vi "RF_calibration_NF_WF1974_scan.vi"() -> ()   [LabVIEW 2017]
uses:
  instr.lib/Tektronix TDS 200 1000 2000 Series/Tektronix TDS 200 1000 2000 Series.lvlib
  instr.lib/Keithley 3390/Keithley 3390.lvlib
panel:
  out "Graph 3":cluster{dbl[], dbl[]}(graph)={[200.0, 300.0, 300.0, 300.0, 300.0], [0.0544000007, 0.0544000007, 0.0903999954, 0.0903999954, 0.1011999995]}
  in  "COMMENT":string="TEST"
  out "Graph 2":cluster{dbl[], dbl[]}(graph)={[200.0, 300.0, 300.0, 300.0, 300.0], [1200.0, 1200.0, 2000.0, 2000.0, 2400.0]}
  out "Graph":cluster{dbl[], dbl[]}(graph)={[200.0, 300.0, 300.0, 300.0, 300.0], [160000.0, 160000.0, 160000.0, 160000.0, 160000.0]}
  in  "Tab Control":enum32{"CONFIG", "MAIN", "DIAGNOSIS"}(tab)
  in  "WF1974":refnum<visa-resource-name>="USB0::0x0D4A::0x000E::9260521::INSTR"
  in  "Columns":string[](array[string])=["SF1/SF2", "l (mm)", "FG freq (Hz)", "FG V (mVpp)", "CH1 Monitor (Vpp)", "CH2 VR (Vpp)", "CH2 Antenna (Vpp)"]
  in  "File path":path=path "C:/LabVIEW/DATA/J-PARC_202206/RF_zscans"
  in  "Tektronix":refnum<visa-resource-name>="USB0::0x0699::0x0365::C035183::INSTR"
  out "File ref (calibration)":refnum<file>
  out "Error Out":errorcluster={"status"=FALSE, "code"=1073676290, "source"="NF WF1973_74 Initialize.vi->RF_calibration_NF_WF1974_scan.vi内のVISAイベント有効"}
  in  "Measure":bool
  in  "Vamp lower lim":dbl=0.4 format="%_4f"
  in  "Vamp upper lim":dbl=3000.0 format="%_4f"
  in  "FG reset":bool
  in  "Amplitude (mVpp)":dbl=1200.0 format="%_6f"
  in  "FG Output":bool
  in  "Frequency (Hz)":dbl=160000.0 format="%_8e"
  out "Measurement index":i32
  out "CH 1 measurement":dbl=0.1011999995 format="%_6g"
  out "CH 2 measurement":dbl=3.4600000381 format="%_6g"
  out "CH3 measurement":dbl=0.00208
  in  "L (mm)":dbl=300.0
  in  "SF1 or2?":u32=1
  out "Latest measurements":dbl[][](array[numeric]) format="%_4e"
  out "index":i32[](array[numeric])
  out "error out (Agilent)":errorcluster
  out "error out (Tektronix)":errorcluster
  out "error out (file operation)":errorcluster
  in  "STOP":bool
  # "Z SCAN OF THE RF FIELD"
  # "SCAN INPUTS"
  # "FG CONTROL"
  # "TEKTRONIX READOUT"
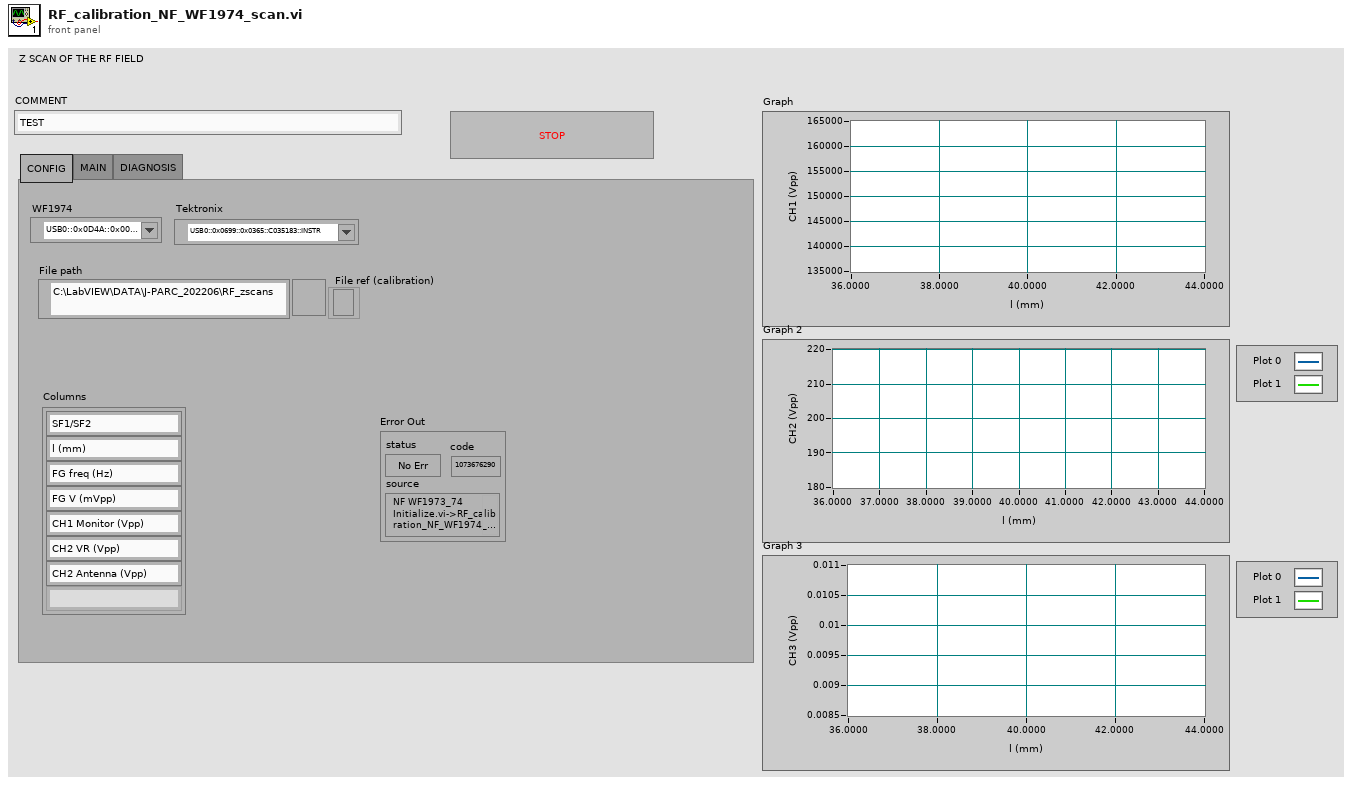
[diagram p1: front panel]
types:
  T1 = cluster{"Baud Rate":u32, "Parity":u16, "Stop Bits":u16, "Flow Control":u16}
  T2 = enum16{"open", "replace", "create", "open or create", "replace or create", "replace or create with confirmation"}
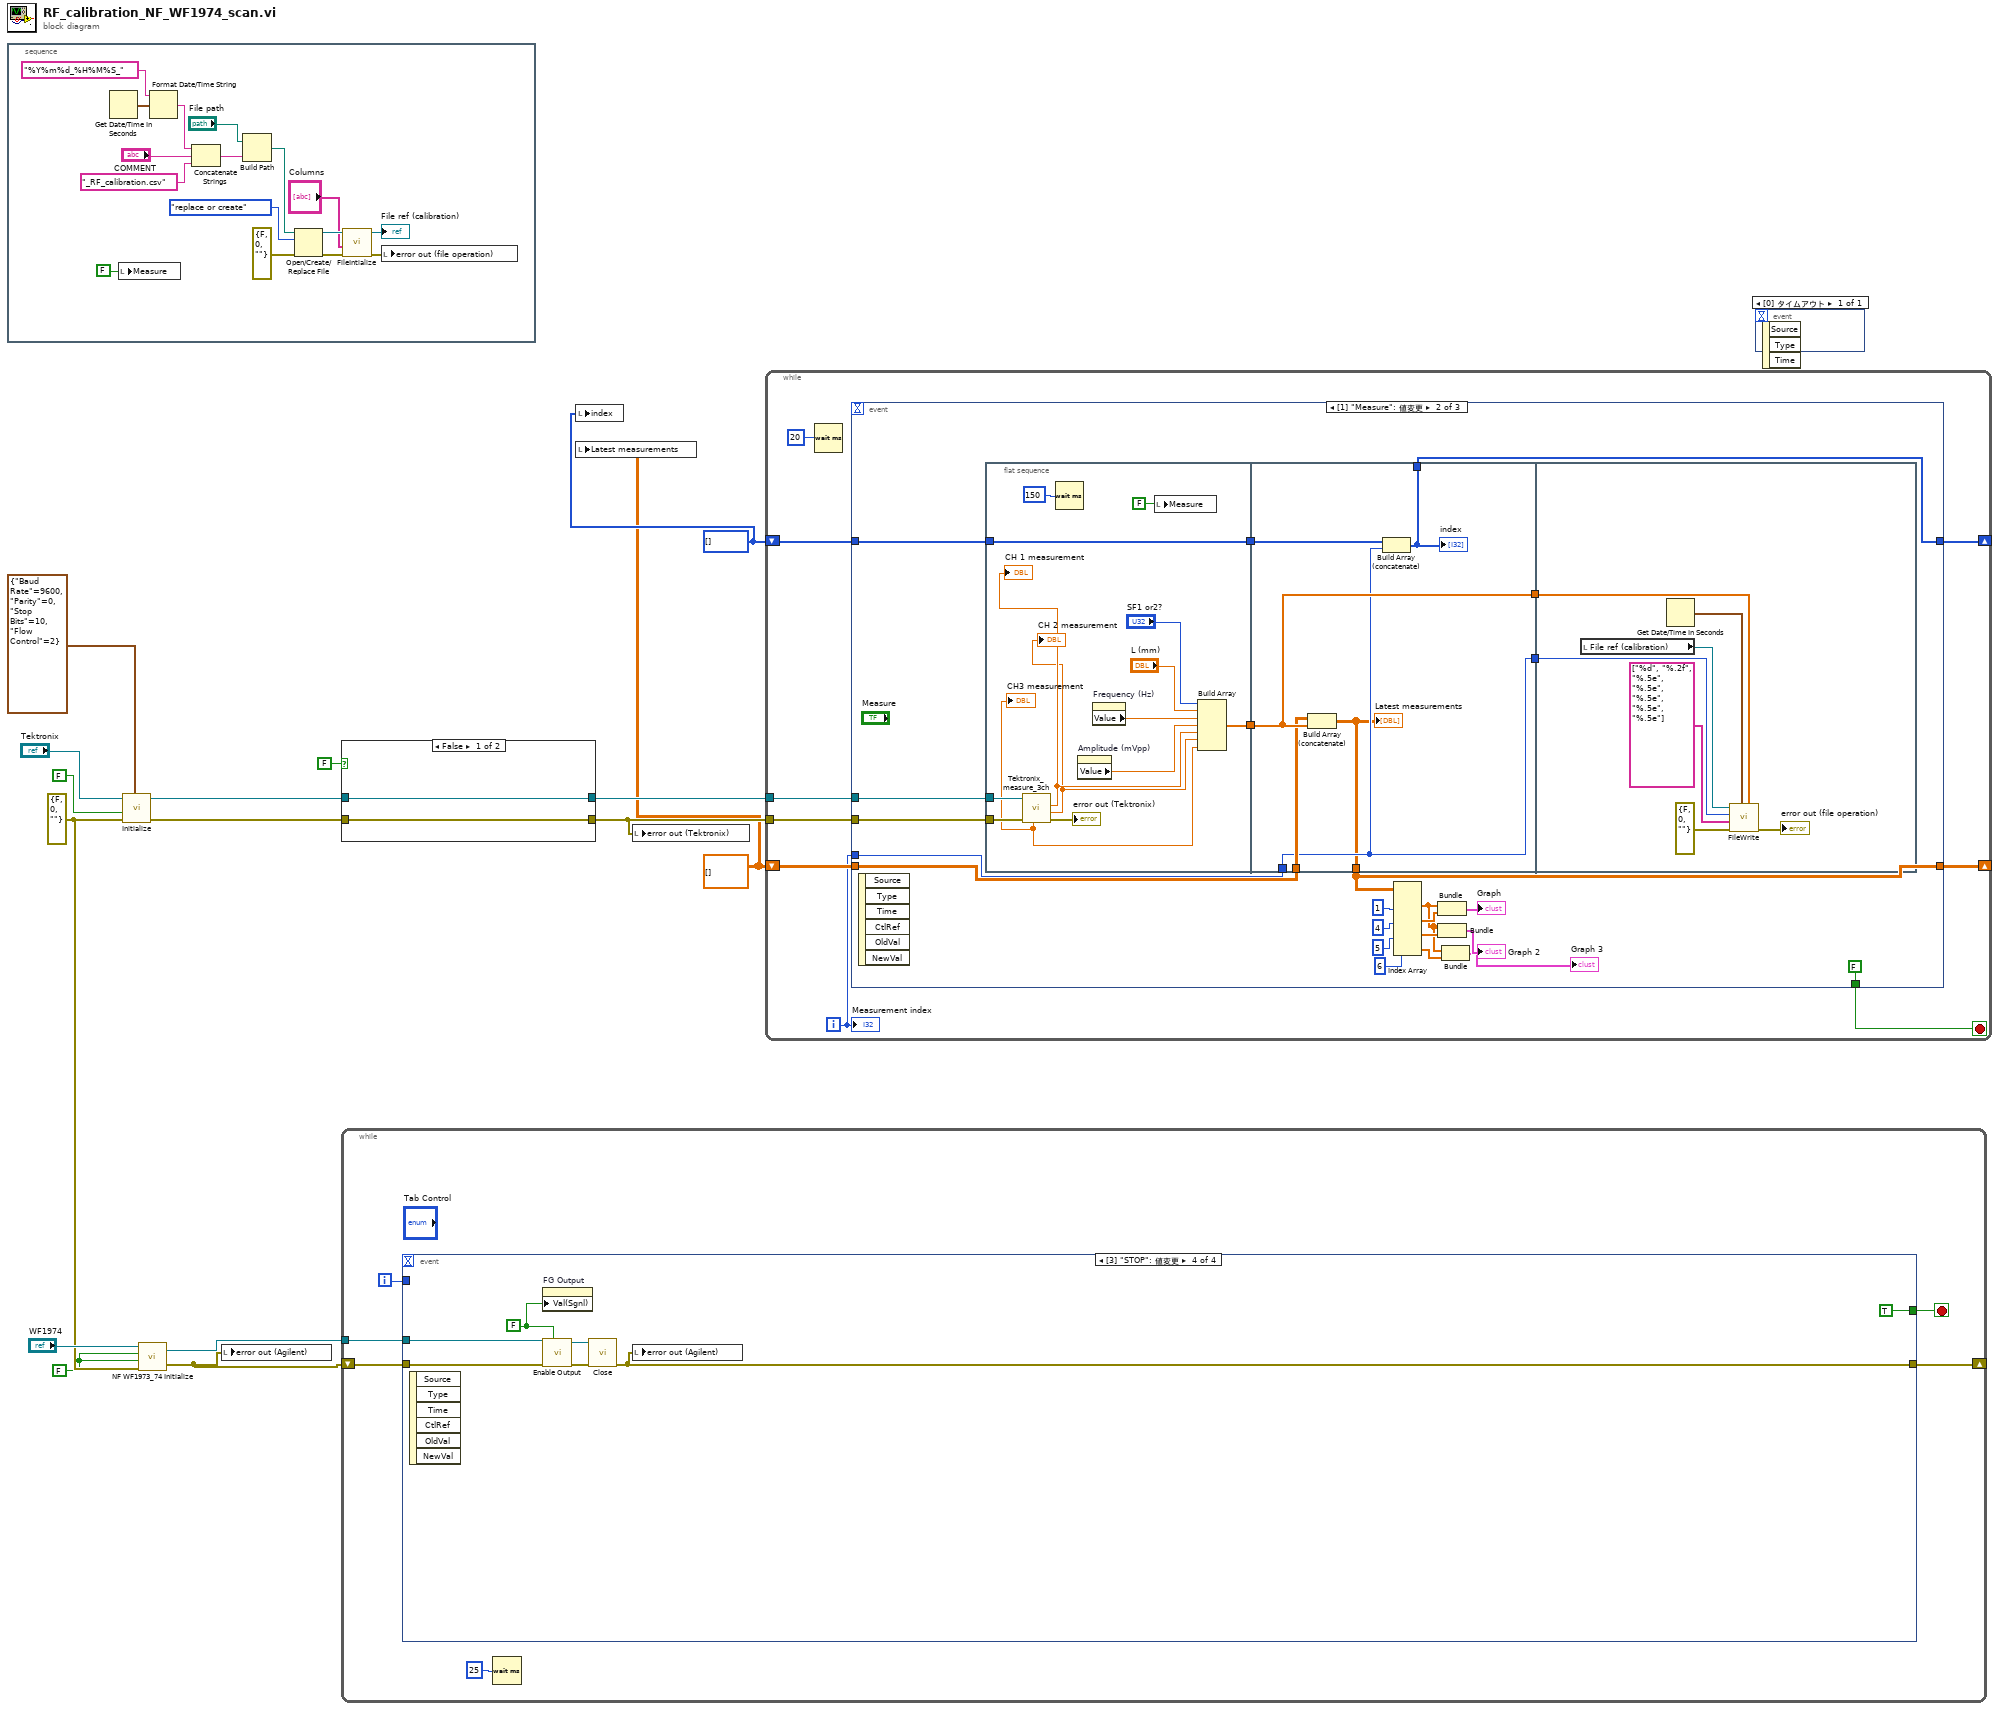
[diagram p0: block diagram]
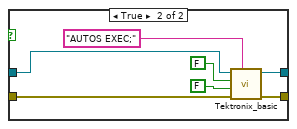
[diagram p2: hidden frame]
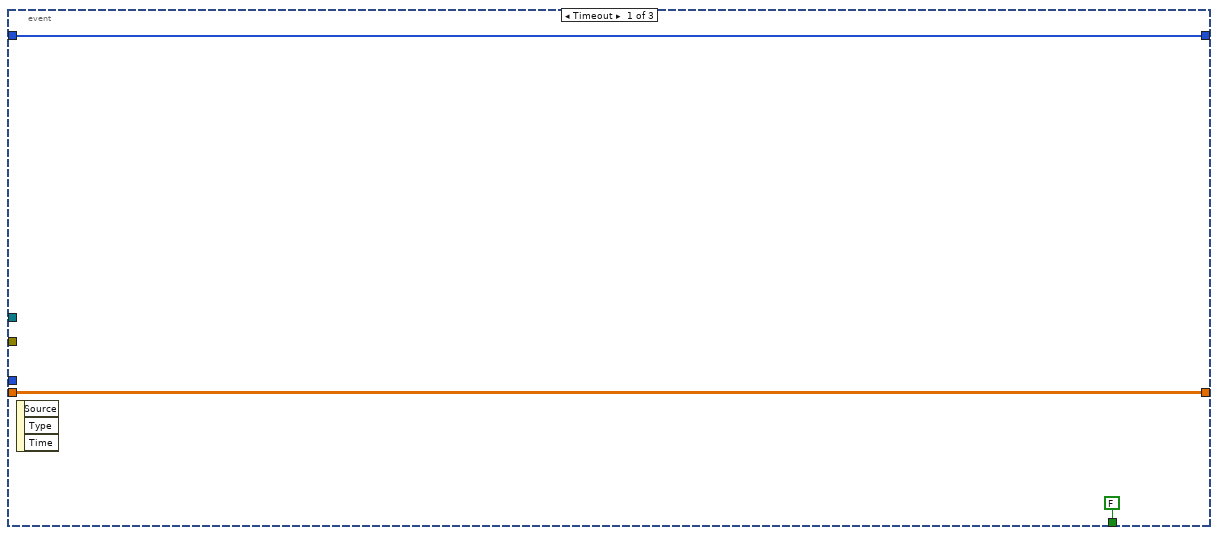
[diagram p3: hidden frame]
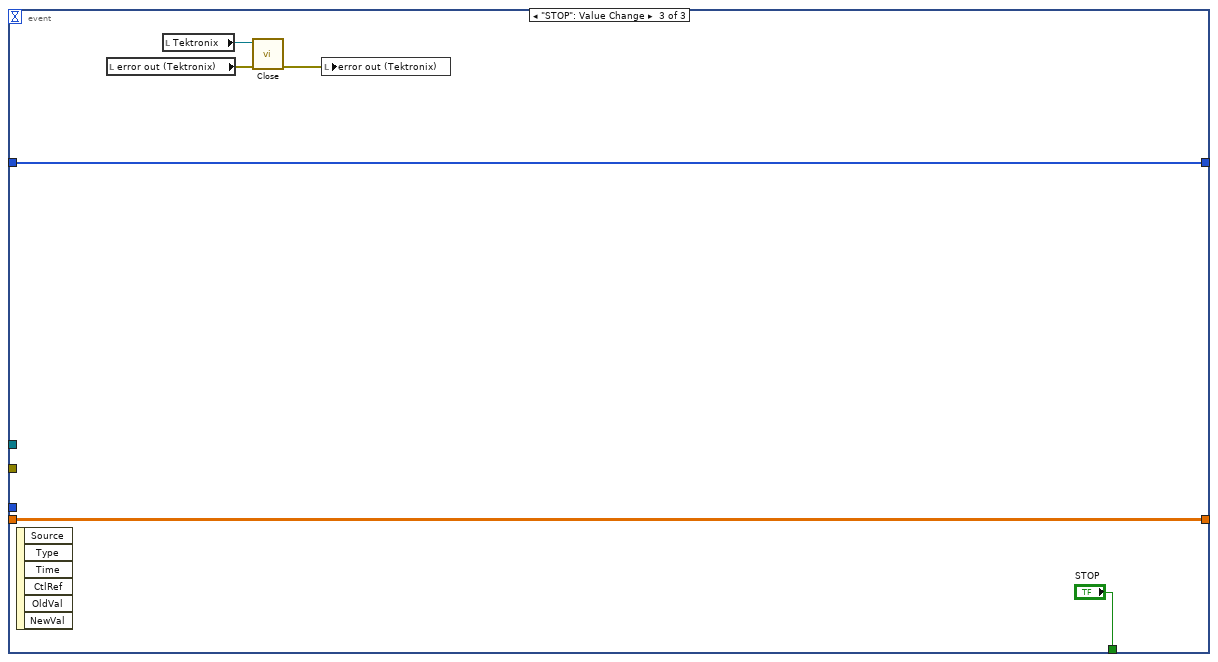
[diagram p4: hidden frame]
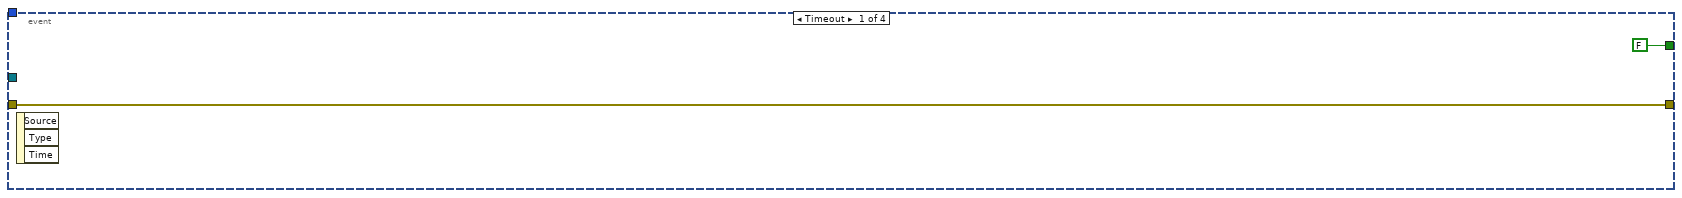
[diagram p5: hidden frame]
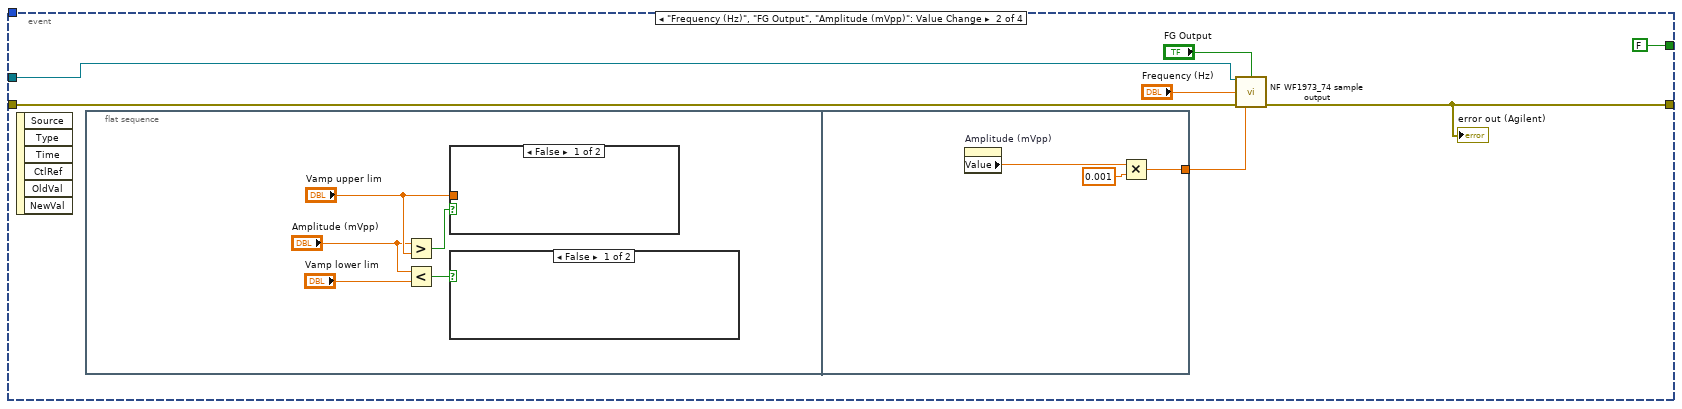
[diagram p6: hidden frame]
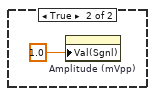
[diagram p7: hidden frame]
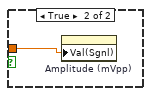
[diagram p8: hidden frame]
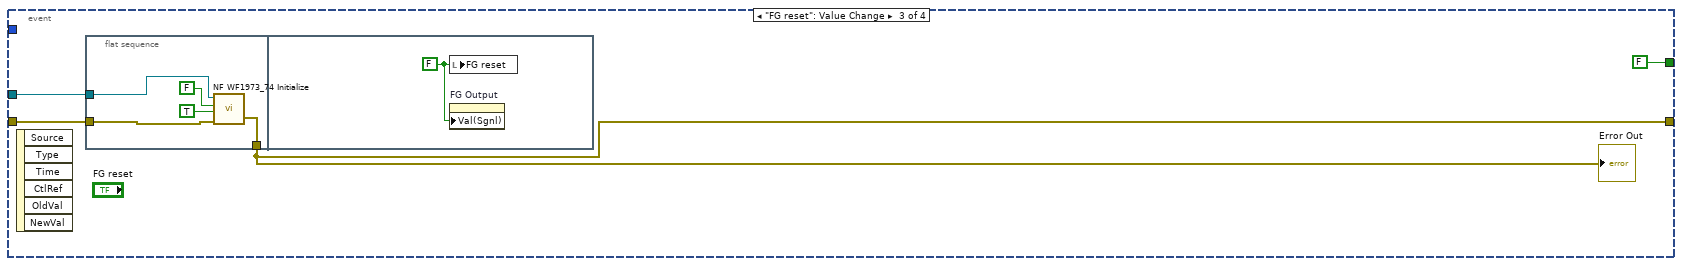
[diagram p9: hidden frame]
diagram:
  w1 = dbl[][] []
  w2 = i32[] []
  w3 = FALSE ("Reset (True)")
  w6 = errorcluster {"status"=FALSE, "code"=0, "source"=""} ("error in (no error)")
  n1 = stacked-sequence {
    frame #0 {
      n2 = Get Date/Time In Seconds() -> (seconds since 1Jan1904=w20:timestamp)
      n3 = local write "Measure"(FALSE ("Measure")) -> ()
      n4 = Format Date/Time String(time format string (%c)="%Y%m%d_%H%M%S_", seconds (now)=w20) -> (date/time string=w18:string)  [unwired: 1 in]
      n5 = Concatenate Strings(w18, "COMMENT", "_RF_calibration.csv") -> (w31:string)
      n6 = Build Path(base path="File path", name or relative path=w31) -> (appended path=w30:path)
      n7 = Open/Create/Replace File(file path (use dialog)=w30, error in=errorcluster {"status"=FALSE, "code"=0, "source"=""}, operation (0:open)=T2."replace or create") -> (refnum out=w27:refnum<file>, error out=w28:errorcluster)  [unwired: 3 in, 1 out]
      n8 = call "FileIntialize.vi"("Error In"=w28, "Labels"="Columns", "refnum in"=w27) -> ("Error Out"=w17:errorcluster, "File Refnum"=→"File ref (calibration)":refnum<file>)  [unwired: 7 in]
      n9 = local write "error out (file operation)"(w17) -> ()
    }
  }
  n10 = call "Initialize.vi"("Serial Configuration"=T1 {"Baud Rate"=9600, "Parity"=0, "Stop Bits"=10, "Flow Control"=2}, "error in (no error)"=w6, "Reset? (T: Yes)"=FALSE, "VISA resource name"="Tektronix") -> ("error out"=w12:errorcluster, "VISA resource name out"=w11:refnum<visa-resource-name>)  [unwired: 1 in, 5 out]
  n11 = call "NF WF1973_74 Initialize.vi"("Error In"=w6, "Reset(T)"=w3, "ID Check(T)"=w3, "VISAsession"="WF1974") -> ("Error Out"=w5:errorcluster, "CopyVISAsession"=w4:refnum<visa-resource-name>)
  n12 = local write "error out (Agilent)"(w5) -> ()
  n13 = case shown="FALSE" FALSE {
    tunnel: w12 -> [w32 w40]
    tunnel: w11 -> [w33 w39]
    tunnel: [w33 w38] -> w10
    tunnel: [w32 w37] -> w9
    frame False {
    }
    frame True {
      n14 = call "Tektronix_basic.vi"("write buffer"="AUTOS EXEC;", "error in (no error)"=w40, "Query?"=FALSE, "Error query?"=FALSE, "VISA resource name"=w39) -> ("error out"=w37:errorcluster, "VISA resource name out"=w38:refnum<visa-resource-name>)  [unwired: 4 in, 1 out]
    }
  }
  n15 = while {
    tunnel: w4 -> [w46]
    shift-right: [w43] -> _
    shift-left: w5 -> [w42]
    i -> [w41]
    stop <- w44 stop-if-true
    n16 = event shown="[3] \"STOP\": 値変更" {
      selector: _ -> [_ _ _ _]
      dyn-events: _ -> [_ _ _ _]
      timeout: _ -> [_ _ _ _]
      tunnel: w46 -> [_ w54 w68 w81]
      tunnel: w42 -> [w47 w53 w67 w77]
      tunnel: [FALSE FALSE FALSE TRUE] -> w44
      tunnel: [w47 w49 w66 w76] -> w43
      tunnel: w41 -> [_ _ _ _]
      event Timeout {
        n17 = event-data() -> ()  [unwired: 1 in, 3 out]
      }
      event "Frequency (Hz)", "FG Output", "Amplitude (mVpp)": Value Change {
        n18 = event-data() -> ()  [unwired: 1 in, 6 out]
        n19 = flat-sequence {
          tunnel: [w64] -> w50
          frame #0 {
            n20 = Greater?(x="Amplitude (mVpp)", y="Vamp upper lim") -> (0:w59:bool)
            n21 = Less?(x="Amplitude (mVpp)", y="Vamp lower lim") -> (x < y?=w56:bool)
            n22 = case shown="FALSE" w59 {
              tunnel: "Vamp upper lim" -> [_ w62]
              frame False {
              }
              frame True {
                n23 = property on="Amplitude (mVpp)" class="DigNum （指定）"("Val(Sgnl)"=w62) -> ()  [unwired: 2 in, 2 out]
              }
            }
            n24 = case shown="FALSE" w56 {
              frame False {
              }
              frame True {
                n25 = property on="Amplitude (mVpp)" class="DigNum （指定）"("Val(Sgnl)"=1.0 ("Value (Signaling)")) -> ()  [unwired: 2 in, 2 out]
              }
            }
          }
          frame #1 {
            n26 = property on="Amplitude (mVpp)" class="DigNum （指定）"() -> ("Value"=w63:dbl)  [unwired: 2 in, 2 out]
            n27 = Multiply(x=w63, y=0.001) -> (x*y=w64:dbl)
          }
        }
        n28 = call "NF WF1973_74 sample output.vi"("VISAsession"=w54, "OUTPUT?(OFF)"="FG Output", "Frequency(1)"="Frequency (Hz)", "error in (no error)"=w53, "Amplitude(1)"=w50) -> ("error out"=w49:errorcluster)  [unwired: 9 in, 1 out]
        "error out (Agilent)" <- w49
      }
      event "FG reset": Value Change {
        n29 = event-data() -> ()  [unwired: 1 in, 6 out]
        n30 = flat-sequence {
          tunnel: w67 -> [w71]
          tunnel: w68 -> [w74]
          tunnel: [w70] -> w66
          frame #0 {
            n31 = call "NF WF1973_74 Initialize.vi"("Error In"=w71, "Reset(T)"=TRUE, "ID Check(T)"=FALSE ("ID Query (True)"), "VISAsession"=w74) -> ("Error Out"=w70:errorcluster)  [unwired: 1 out]
          }
          frame #1 {
            w75 = FALSE ("Value (Signaling)")
            n32 = local write "FG reset"(w75) -> ()
            n33 = property on="FG Output" class="Bool （指定）"("Val(Sgnl)"=w75) -> ()  [unwired: 2 in, 2 out]
          }
        }
        "Error Out" <- w66
      }
      event "STOP": Value Change {
        w79 = FALSE ("Enable Output  (T: Enable)")
        n34 = event-data() -> ()  [unwired: 1 in, 6 out]
        n35 = property on="FG Output" class="Bool （指定）"("Val(Sgnl)"=w79) -> ()  [unwired: 2 in, 2 out]
        n36 = call "Enable Output.vi"("Enable Output (T: Enable)"=w79, "error in (no error)"=w77, "VISA resource name"=w81) -> ("error out"=w80:errorcluster, "VISA resource name out"=w82:refnum<visa-resource-name>)  [unwired: 7 in]
        n37 = call "Close.vi"("error in (no error)"=w80, "VISA resource name"=w82) -> ("error out"=w76:errorcluster)  [unwired: 9 in]
        n38 = local write "error out (Agilent)"(w76) -> ()
      }
    }
    n39 = Wait (ms)(milliseconds to wait=u32 25) -> ()  [unwired: 1 out]
  }
  n40 = local write "index"(w2) -> ()
  n41 = local write "Latest measurements"(w1) -> ()
  n42 = local write "error out (Tektronix)"(w9) -> ()
  n43 = while {
    tunnel: w9 -> [w91]
    tunnel: w10 -> [w90]
    shift-right: [w89] -> _
    shift-left: w2 -> [w88]
    shift-right: [w87] -> _
    shift-left: w1 -> [w86]
    i -> [w85]
    stop <- w83 stop-if-true
    n44 = Wait (ms)(milliseconds to wait=u32 20) -> ()  [unwired: 1 out]
    n45 = event shown="[1] \"Measure\": 値変更" {
      selector: _ -> [_ _ _]
      dyn-events: _ -> [_ _ _]
      timeout: _ -> [_ _ _]
      tunnel: w91 -> [_ w116 _]
      tunnel: w90 -> [_ w115 _]
      tunnel: [w94 w111 w147] -> w89
      tunnel: w88 -> [w94 w117 w147]
      tunnel: [w93 w112 w146] -> w87
      tunnel: w86 -> [w93 w113 w146]
      tunnel: w85 -> [_ w114 _]
      tunnel: [FALSE ("STOP") FALSE ("STOP") "STOP"] -> w83
      event Timeout {
        n46 = event-data() -> ()  [unwired: 1 in, 3 out]
      }
      event "Measure": Value Change {
        n47 = event-data() -> ()  [unwired: 1 in, 6 out]
        n48 = flat-sequence {
          tunnel: [w131] -> w110
          tunnel: w117 -> [w131]
          tunnel: w116 -> [w125]
          tunnel: w115 -> [w124]
          tunnel: [w123] -> w109
          tunnel: w110 -> [w136]
          tunnel: [w137] -> w108
          tunnel: w109 -> [w137]
          tunnel: w114 -> [w134]
          tunnel: w113 -> [w135]
          tunnel: [w132] -> w112
          tunnel: [w134] -> w107
          tunnel: [w133] -> w111
          tunnel: w108 -> [w139]
          tunnel: w107 -> [w138]
          frame #0 {
            n49 = call "Tektronix_measure_3ch.vi"("error in (no error)"=w125, "VISA resource name"=w124) -> ("error out"=→"error out (Tektronix)":errorcluster, "Measurement 2"=w119:dbl, "Measurement 1"=w120:dbl, "Measurement 3"=w118:dbl)  [unwired: 2 in, 4 out]
            "CH 1 measurement" <- w120
            "CH 2 measurement" <- w119
            "CH3 measurement" <- w118
            n50 = Wait (ms)(milliseconds to wait=u32 150) -> ()  [unwired: 1 out]
            n51 = property on="Amplitude (mVpp)" class="DigNum （指定）"() -> ("Value"=w127:dbl)  [unwired: 2 in, 2 out]
            n52 = property on="Frequency (Hz)" class="DigNum （指定）"() -> ("Value"=w126:dbl)  [unwired: 2 in, 2 out]
            n53 = local write "Measure"(FALSE ("Measure")) -> ()
            n54 = Build Array("SF1 or2?", "L (mm)", w126, w127, w120, w119, w118) -> (w123:dbl[])
          }
          frame #1 {
            n55 = Build Array (concatenate)(w135, w137) -> (w132:dbl[][])
            "Latest measurements" <- w132
            n56 = Build Array (concatenate)(w136, w134) -> (w133:i32[])
            "index" <- w133
          }
          frame #2 {
            n57 = local read "File ref (calibration)"() -> (w144:refnum<file>)
            n58 = Get Date/Time In Seconds() -> (seconds since 1Jan1904=w141:timestamp)
            n59 = call "FileWrite.vi"("DataArray"=w139, "Time Stamp"=w141, "Error In"=errorcluster {"status"=FALSE, "code"=0, "source"=""}, "FileFormat"=string[] ["%d", "%.2f", "%.5e", "%.5e", "%.5e", "%.5e", "%.5e"], "Index"=w138, "refnum in"=w144) -> ("Error Out"=→"error out (file operation)":errorcluster)  [unwired: 4 in, 1 out]
          }
        }
        n60 = Index Array(array=w112, index (col) #1=1 ("無効な指標 （列）"), index (col) #2=4 ("disabled index (col)"), index (col) #3=5 ("index (row)"), index (col) #4=6 ("指標 （列）")) -> (element #1=w98:dbl[], element #2=w103:dbl[], element #3=w101:dbl[], element #4=w97:dbl[])  [unwired: 4 in]
        n61 = Bundle(w98, w103) -> (→"Graph":cluster{dbl[], dbl[]})  [unwired: 1 in]
        n62 = Bundle(w98, w101) -> (→"Graph 2":cluster{dbl[], dbl[]})  [unwired: 1 in]
        n63 = Bundle(w98, w97) -> (→"Graph 3":cluster{dbl[], dbl[]})  [unwired: 1 in]
      }
      event "STOP": Value Change {
        n64 = event-data() -> ()  [unwired: 1 in, 6 out]
        n65 = local read "error out (Tektronix)"() -> (w149:errorcluster)
        n66 = local read "Tektronix"() -> (w148:refnum<visa-resource-name>)
        n67 = call "Close.vi"("error in (no error)"=w149, "VISA resource name"=w148) -> ("error out"=w150:errorcluster)  [unwired: 9 out]
        n68 = local write "error out (Tektronix)"(w150) -> ()
      }
    }
    "Measurement index" <- w85
  }
  n69 = event shown="[0] タイムアウト" {
    selector: _ -> [_]
    dyn-events: _ -> [_]
    timeout: _ -> [_]
    event Timeout {
      n70 = event-data() -> ()  [unwired: 1 in, 3 out]
    }
  }
